vi "Expiry String.vi"(10 "As Max-Age? (T)":bool=TRUE, 11 "Time Stamp":timestamp) -> (2 "Set?":bool, 3 "String":string)   [LabVIEW 2020, in "HTTP Utils.lvlib" / "Cookie.lvclass"]
uses:
  Cookie.lvclass
  Cookie.lvclass/Cookie.ctl
  HTTP Utils.lvlib
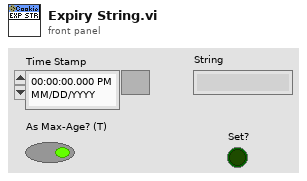
[diagram p1: front panel]
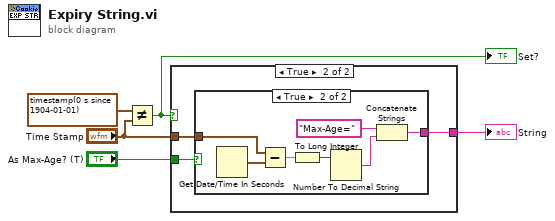
[diagram p0: block diagram]
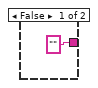
[diagram p2: hidden frame]
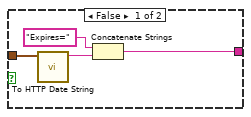
[diagram p3: hidden frame]
diagram:
  n1 = Not Equal?(x=timestamp(0 s since 1904-01-01), y="Time Stamp") -> (x != y?=w1:bool)
  "Set?" <- w1
  n2 = case shown="True" w1 {
    tunnel: "Time Stamp" -> [_ w9]
    tunnel: "As Max-Age? (T)" -> [_ w8]
    tunnel: ["" w7] -> w2
    frame False {
    }
    frame True {
      n3 = case shown="True" w8 {
        tunnel: w9 -> [w13 w19]
        tunnel: [w11 w14] -> w7
        frame False {
          n4 = call "To HTTP Date String.vi"("Time Stamp"=w13) -> ("HTTP Date"=w12:string)  [unwired: 10 in]
          n5 = Concatenate Strings("Expires=", w12) -> (w11:string)
        }
        frame True {
          n6 = Get Date/Time In Seconds() -> (seconds since 1Jan1904=w20:timestamp)
          n7 = Subtract(x=w19, y=w20) -> (x-y=w18:dbl)
          n8 = To Long Integer(number=w18) -> (32bit integer=w17:i32)
          n9 = Number To Decimal String(number=w17) -> (decimal integer string=w15:string)  [unwired: 1 in]
          n10 = Concatenate Strings("Max-Age=" ("format string"), w15) -> (w14:string)
        }
      }
    }
  }
  "String" <- w2
